vi "Page_Advanced_Initialize.vi"(6 "ctl references":T1, 8 "error in (no error)":errorcluster, 11 "AB_DepDLL in":refnum<class "AB_DepDLL.lvclass">) -> (0 "error out":errorcluster, 3 "AB_DepDLL out":refnum<class "AB_DepDLL.lvclass">)   [LabVIEW 2020, in "AB_DepDLL.lvclass"]
uses:
  <vilib>/AppBuilder/AB_Classes/DepDLL/AB_DepDLL.lvclass
  <resource>/Framework/Providers/Builds/AppBuilder/AB_UI_Page_Advanced_References.ctl
  <vilib>/AppBuilder/AB_Classes/DLL/AB_DLL.lvclass
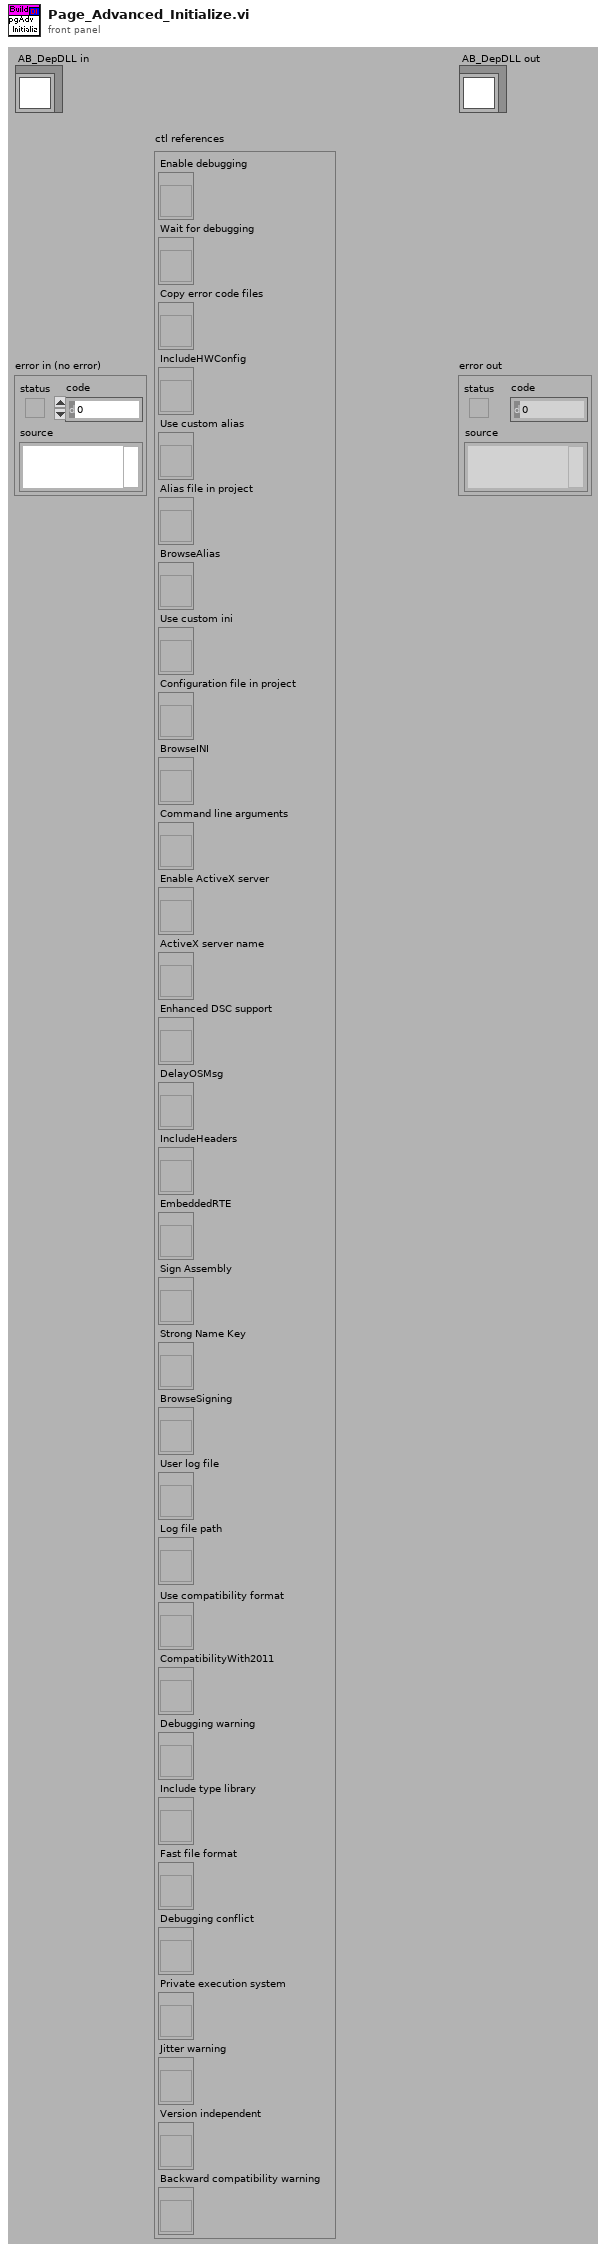
[diagram p1: front panel]
types:
  T1 = typedef "AB_UI_Page_Advanced_References.ctl" = cluster{"Enable debugging":refnum<vi>, "Wait for debugging":refnum<vi>, "Copy error code files":refnum<vi>, "IncludeHWConfig":refnum<vi>, "Use custom alias":refnum<vi>, "Alias file in project":refnum<vi>, "BrowseAlias":refnum<vi>, "Use custom ini":refnum<vi>, "Configuration file in project":refnum<vi>, "BrowseINI":refnum<vi>, "Command line arguments":refnum<vi>, "Enable ActiveX server":refnum<vi>, "ActiveX server name":refnum<vi>, "Enhanced DSC support":refnum<vi>, "DelayOSMsg":refnum<vi>, "IncludeHeaders":refnum<vi>, "EmbeddedRTE":refnum<vi>, "Sign Assembly":refnum<vi>, "Strong Name Key":refnum<vi>, "BrowseSigning":refnum<vi>, "User log file":refnum<vi>, "Log file path":refnum<vi>, "Use compatibility format":refnum<vi>, "CompatibilityWith2011":refnum<vi>, "Debugging warning":refnum<vi>, "Include type library":refnum<vi>, "Fast file format":refnum<vi>, "Debugging conflict":refnum<vi>, "Private execution system":refnum<vi>, "Jitter warning":refnum<vi>, "Version independent":refnum<vi>, "Backward compatibility warning":refnum<vi>}
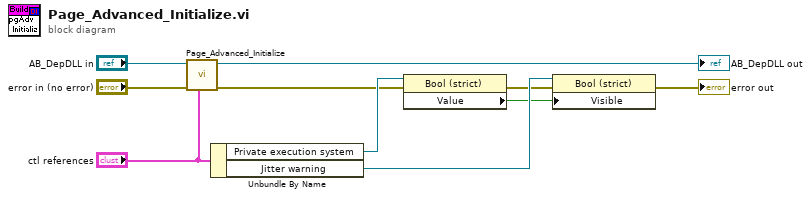
[diagram p0: block diagram]
diagram:
  n1 = call-parent "Page_Advanced_Initialize.vi"("ctl references"="ctl references", "error in (no error)"="error in (no error)", "AB_DLL in"="AB_DepDLL in") -> ("error out"=w3:errorcluster, "AB_DLL out"=→"AB_DepDLL out":refnum<class "AB_DepDLL.lvclass">)  [unwired: 7 in]
  n2 = Unbundle By Name("ctl references") -> ("Private execution system"=w6:refnum<vi>, "Jitter warning"=w5:refnum<vi>)
  n3 = property class="Bool (strict)"(reference=w6, error in=w3) -> (error out=w4:errorcluster, "Value"=w1:bool)  [unwired: 1 out]
  n4 = property class="Bool (strict)"(reference=w5, error in=w4, "Visible"=w1) -> (error out=→"error out":errorcluster)  [unwired: 1 out]
